vi "find tag.vi"(10 "tag":refnum<class "tag descriptor.lvclass">, 11 "tags in":refnum<class "tag descriptor.lvclass">[](array[class])) -> (3 "index":i32)   [LabVIEW 2013, in "tag bus.lvlib" / "tag descriptor.lvclass"]
doc: "Locates a specific tag by name in the provided list of tags."
uses:
  tag descriptor.lvclass
  tag descriptor.lvclass/tag descriptor.ctl
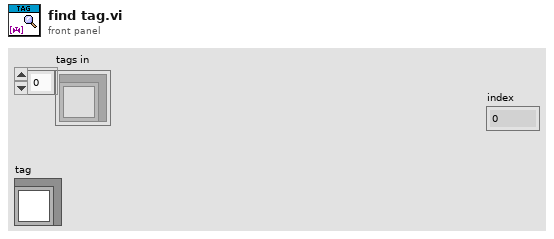
[diagram p1: front panel]
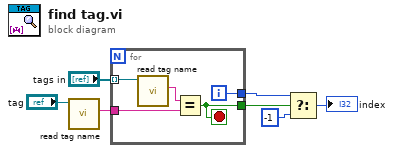
[diagram p0: block diagram]
diagram:
  n1 = call "read tag name.vi"("system tag in"="tag") -> ("name"=w1:string)  [unwired: 8 in, 2 out]
  n2 = for {
    tunnel: "tags in" -> [w12] mode=indexing
    tunnel: w1 -> [w10]
    tunnel: [w9] -> w6
    tunnel: [w8] -> w5
    i -> [w8]
    stop <- w9 stop-if-true
    n3 = call "read tag name.vi"("system tag in"=w12) -> ("name"=w11:string)  [unwired: 8 in, 2 out]
    n4 = Equal?(x=w11, y=w10) -> (x = y?=w9:bool)
  }
  n5 = Select(t=w5, s=w6, f=-1) -> (s? t:f=→"index":i32)
